vi "CPF_accurate.vi"(1 "y":dbl=1.0, 2 "x":dbl=1.0) -> (0 "CPF Value":cdb=0.30474420525691914+0.2082189382028327i format="%#_12g")   [LabVIEW 2015]
panel:
  # "CPF algorithm"
  # "Accurate CPF algorithm (default):\n  Computes the complex probability function using a rational series with 42\n  terms. It is assumed that Im(z) > 0 or Im(z) = 0. (Source: \n  jstor.org/stable/2158232). A series was simplified to 37 terms introducing\n  less than 10^(-17) deviations on mHT profile.\n\nStandard Input Parameters:\n-------------------- \nx  : Real part of input complex parameter\ny  : Imaginary part of input complex parameter\n\nThe function has one output:\n--------------------\n(1): Complex probability function"
  # "Output Section"
  # "Input Section"
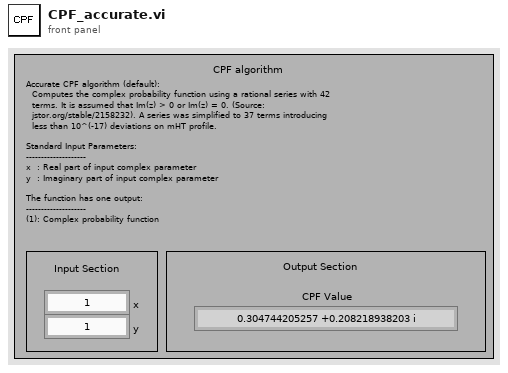
[diagram p1: front panel]
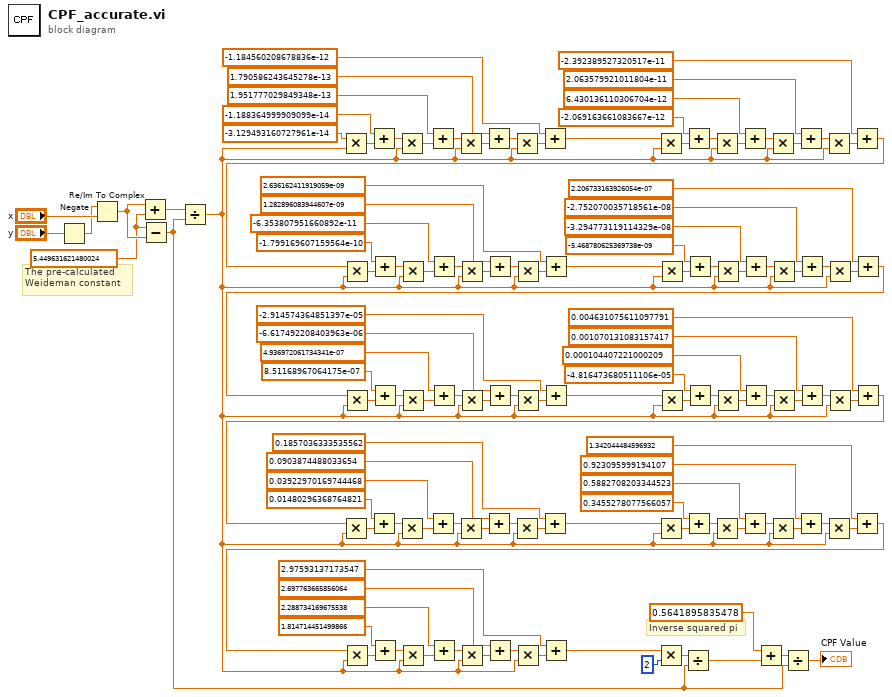
[diagram p0: block diagram]
diagram:
  w118 = 5.449631621480024 ("L")
  # "Inverse squared pi"
  # "The pre-calculated \nWeideman constant"
  n1 = Negate(x="y") -> (-x=w120:dbl)
  n2 = Re/Im To Complex(1:"x", 2:w120) -> (0:w119:cdb)
  n3 = Add(x=w119, y=w118) -> (x+y=w117:cdb)
  n4 = Subtract(x=w118, y=w119) -> (x-y=w109:cdb)
  n5 = Divide(x=w117, y=w109) -> (x/y=w116:cdb)
  n6 = Multiply(x=-3.129493160727961e-14, y=w116) -> (x*y=w108:cdb)
  n7 = Add(x=-1.188364999909099e-14, y=w108) -> (x+y=w107:cdb)
  n8 = Multiply(x=w107, y=w116) -> (x*y=w105:cdb)
  n9 = Add(x=1.951777029849348e-13, y=w105) -> (x+y=w106:cdb)
  n10 = Multiply(x=w106, y=w116) -> (x*y=w102:cdb)
  n11 = Add(x=1.790586243645278e-13, y=w102) -> (x+y=w104:cdb)
  n12 = Multiply(x=w104, y=w116) -> (x*y=w103:cdb)
  n13 = Add(x=-1.184560208678836e-12, y=w103) -> (x+y=w94:cdb)
  n14 = Multiply(x=w94, y=w116) -> (x*y=w101:cdb)
  n15 = Add(x=-2.069163661083667e-12, y=w101) -> (x+y=w100:cdb)
  n16 = Multiply(x=w100, y=w116) -> (x*y=w98:cdb)
  n17 = Add(x=6.430136110306704e-12, y=w98) -> (x+y=w99:cdb)
  n18 = Multiply(x=w99, y=w116) -> (x*y=w95:cdb)
  n19 = Add(x=2.063579921011804e-11, y=w95) -> (x+y=w97:cdb)
  n20 = Multiply(x=w97, y=w116) -> (x*y=w96:cdb)
  n21 = Add(x=-2.392389527320517e-11, y=w96) -> (x+y=w61:cdb)
  n22 = Multiply(x=w61, y=w116) -> (x*y=w84:cdb)
  n23 = Add(x=-1.799169607159564e-10, y=w84) -> (x+y=w83:cdb)
  n24 = Multiply(x=w83, y=w116) -> (x*y=w81:cdb)
  n25 = Add(x=-6.353807951660892e-11, y=w81) -> (x+y=w82:cdb)
  n26 = Multiply(x=w82, y=w116) -> (x*y=w78:cdb)
  n27 = Add(x=1.282896083944607e-09, y=w78) -> (x+y=w80:cdb)
  n28 = Multiply(x=w80, y=w116) -> (x*y=w79:cdb)
  n29 = Add(x=2.636162411919059e-09, y=w79) -> (x+y=w70:cdb)
  n30 = Multiply(x=w70, y=w116) -> (x*y=w77:cdb)
  n31 = Add(x=-5.468780625369738e-09, y=w77) -> (x+y=w76:cdb)
  n32 = Multiply(x=w76, y=w116) -> (x*y=w74:cdb)
  n33 = Add(x=-3.294773119114329e-08, y=w74) -> (x+y=w75:cdb)
  n34 = Multiply(x=w75, y=w116) -> (x*y=w71:cdb)
  n35 = Add(x=-2.752070035718561e-08, y=w71) -> (x+y=w73:cdb)
  n36 = Multiply(x=w73, y=w116) -> (x*y=w72:cdb)
  n37 = Add(x=2.206733163926054e-07, y=w72) -> (x+y=w37:cdb)
  n38 = Multiply(x=w37, y=w116) -> (x*y=w60:cdb)
  n39 = Add(x=8.51168967064175e-07, y=w60) -> (x+y=w59:cdb)
  n40 = Multiply(x=w59, y=w116) -> (x*y=w57:cdb)
  n41 = Add(x=4.936972061734341e-07, y=w57) -> (x+y=w58:cdb)
  n42 = Multiply(x=w58, y=w116) -> (x*y=w54:cdb)
  n43 = Add(x=-6.617492208403963e-06, y=w54) -> (x+y=w56:cdb)
  n44 = Multiply(x=w56, y=w116) -> (x*y=w55:cdb)
  n45 = Add(x=-2.914574364851397e-05, y=w55) -> (x+y=w46:cdb)
  n46 = Multiply(x=w46, y=w116) -> (x*y=w53:cdb)
  n47 = Add(x=-4.816473680511106e-05, y=w53) -> (x+y=w52:cdb)
  n48 = Multiply(x=w52, y=w116) -> (x*y=w50:cdb)
  n49 = Add(x=0.000104407221000209, y=w50) -> (x+y=w51:cdb)
  n50 = Multiply(x=w51, y=w116) -> (x*y=w47:cdb)
  n51 = Add(x=0.001070131083157417, y=w47) -> (x+y=w49:cdb)
  n52 = Multiply(x=w49, y=w116) -> (x*y=w48:cdb)
  n53 = Add(x=0.004631075611097791, y=w48) -> (x+y=w1:cdb)
  n54 = Multiply(x=w1, y=w116) -> (x*y=w36:cdb)
  n55 = Add(x=0.01480296368764821, y=w36) -> (x+y=w35:cdb)
  n56 = Multiply(x=w35, y=w116) -> (x*y=w33:cdb)
  n57 = Add(x=0.03922970169744468, y=w33) -> (x+y=w34:cdb)
  n58 = Multiply(x=w34, y=w116) -> (x*y=w30:cdb)
  n59 = Add(x=0.0903874488033654, y=w30) -> (x+y=w32:cdb)
  n60 = Multiply(x=w32, y=w116) -> (x*y=w31:cdb)
  n61 = Add(x=0.1857036333535562, y=w31) -> (x+y=w22:cdb)
  n62 = Multiply(x=w22, y=w116) -> (x*y=w29:cdb)
  n63 = Add(x=0.3455278077566057, y=w29) -> (x+y=w28:cdb)
  n64 = Multiply(x=w28, y=w116) -> (x*y=w26:cdb)
  n65 = Add(x=0.5882708203344523, y=w26) -> (x+y=w27:cdb)
  n66 = Multiply(x=w27, y=w116) -> (x*y=w23:cdb)
  n67 = Add(x=0.923095999194107, y=w23) -> (x+y=w25:cdb)
  n68 = Multiply(x=w25, y=w116) -> (x*y=w24:cdb)
  n69 = Add(x=1.342044484596932, y=w24) -> (x+y=w2:cdb)
  n70 = Multiply(x=w2, y=w116) -> (x*y=w13:cdb)
  n71 = Add(x=1.814714451499866, y=w13) -> (x+y=w12:cdb)
  n72 = Multiply(x=w12, y=w116) -> (x*y=w10:cdb)
  n73 = Add(x=2.288734169675538, y=w10) -> (x+y=w11:cdb)
  n74 = Multiply(x=w11, y=w116) -> (x*y=w7:cdb)
  n75 = Add(x=2.697763665856064, y=w7) -> (x+y=w9:cdb)
  n76 = Multiply(x=w9, y=w116) -> (x*y=w8:cdb)
  n77 = Add(x=2.97593137173547, y=w8) -> (x+y=w115:cdb)
  n78 = Multiply(x=w115, y=2) -> (x*y=w113:cdb)
  n79 = Divide(x=w113, y=w109) -> (x/y=w112:cdb)
  n80 = Add(x=0.5641895835478, y=w112) -> (x+y=w110:cdb)
  n81 = Divide(x=w110, y=w109) -> (x/y=→"CPF Value":cdb)
